vi "InspectExecuteCleanup.vi"(6 "Error":errorcluster, 7 "Actor":refnum<class "Actor.lvclass">, 9 "PreInspectExecuteError":errorcluster, 10 "Msg":T1 {"MsgAttribs"."AbsoluteTime" format="%<%x %.3X>T"}, 11 "Actor":T6) -> (2 "Msg":T1 {"MsgAttribs"."AbsoluteTime" format="%<%x %.3X>T"}, 3 "Actor":T6, 4 "Error":errorcluster, 5 "Actor":refnum<class "Actor.lvclass">)   [LabVIEW 2020, in "_Template.lvlib" / "{{Actor}}.lvlib" / "Actor.lvclass"]
uses:
  Actor.lvclass
  jettl/jettl/Metadata/Metadata.lvclass
  jettl/jettl/Msg/Msg.lvclass
  Actor.lvclass/Actor.ctl
  jettl/jettl/Actor/Actor.lvclass
  jettl/jettl/Origin.ctl
  jettl/jettl/jettl.lvlib
  jettl/jettl/Lifecycle.ctl
  jettl/jettl/MsgExecuteType.ctl
  jettl/jettl/MsgAttribs.ctl
  jettl/jettl/Msg.ctl
  jettl/jettl/PostSetup.ctl
  jettl/jettl/PreSetup.ctl
  jettl/jettl/MsgNames.ctl
  jettl/jettl/ActorAttribs.ctl
  jettl/jettl/ChildActors.ctl
  jettl/jettl/Actor.ctl
panel:
  # "This front panel should not be manipulated."
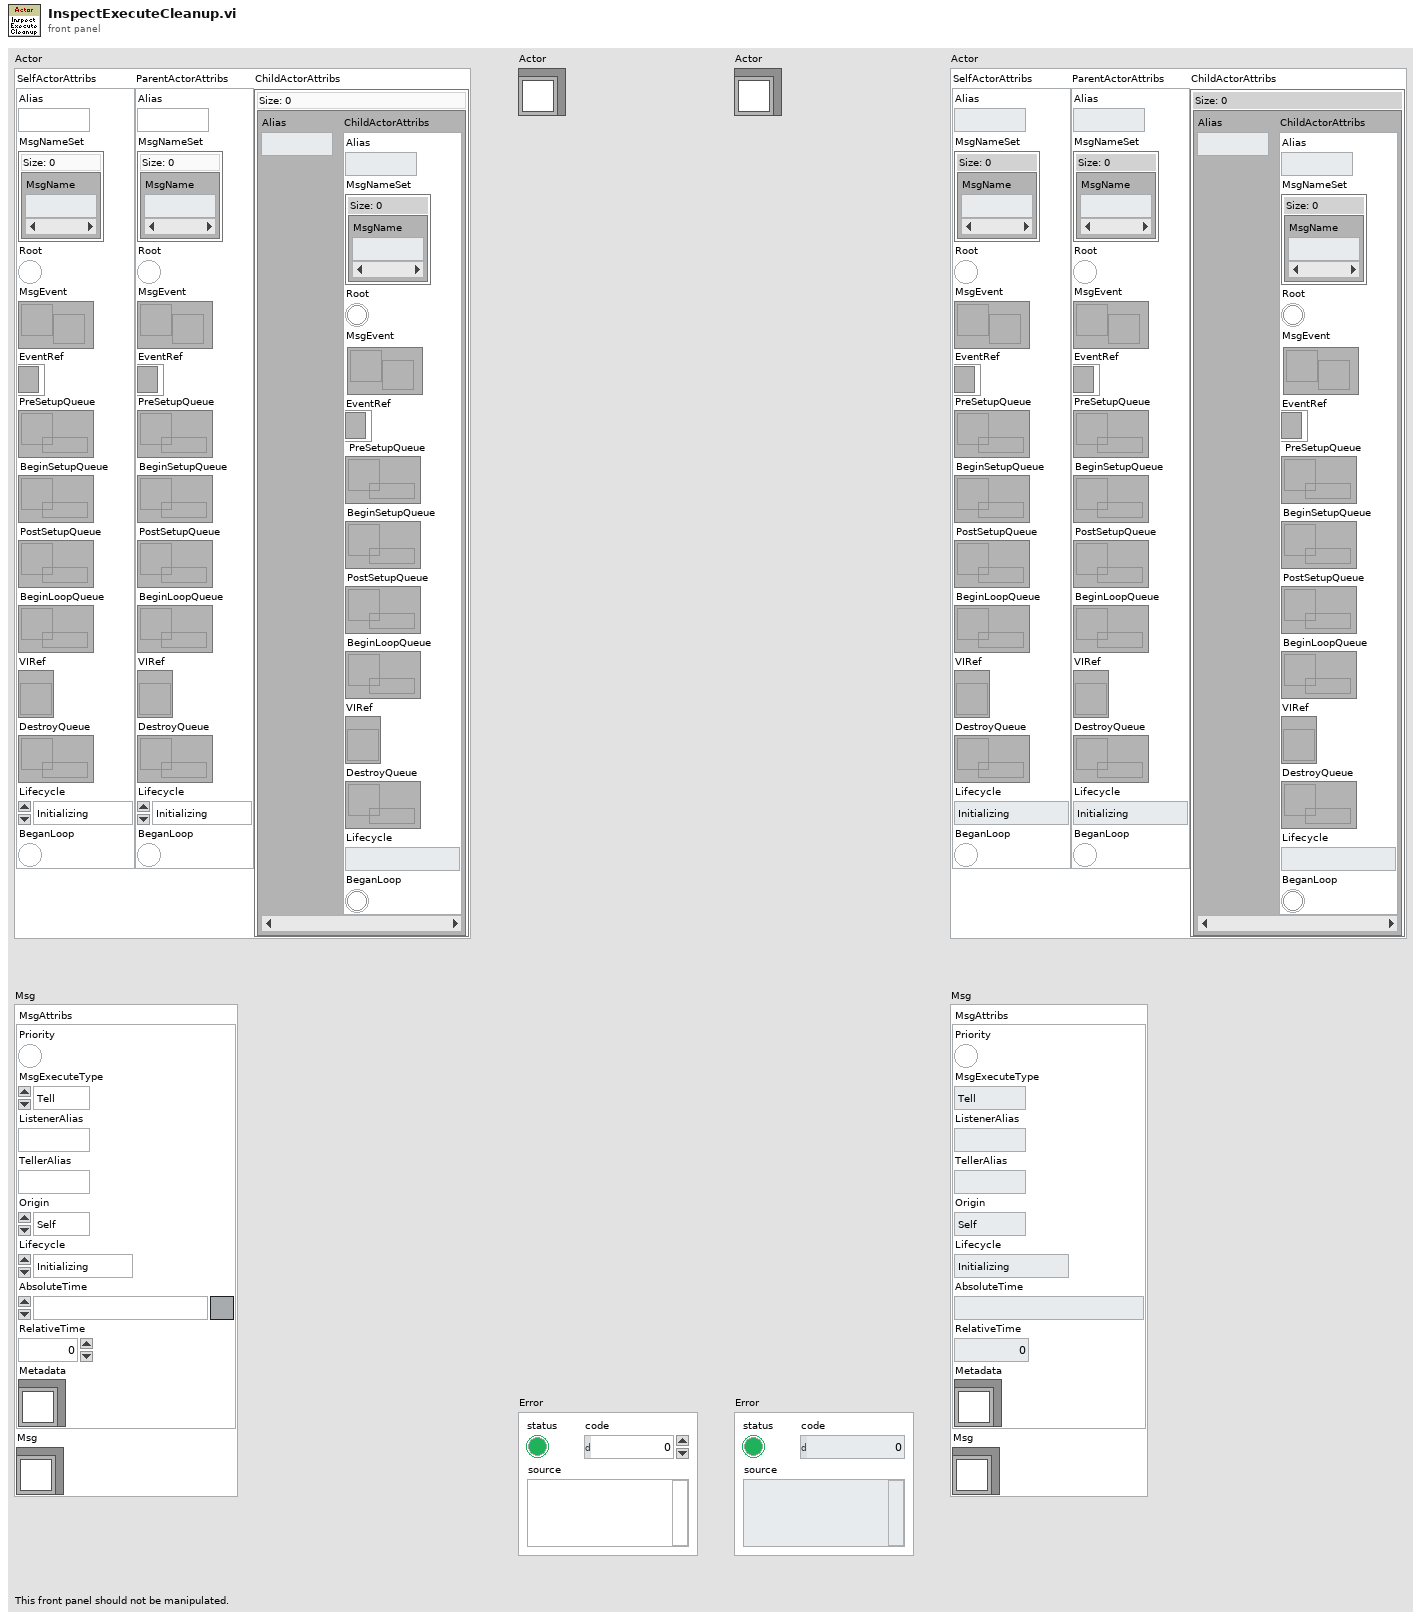
[diagram p1: front panel]
types:
  T1 = typedef "jettl.lvlib/Msg.ctl" = cluster{"MsgAttribs":T2, "Msg":refnum<class "Msg.lvclass">}
  T2 = typedef "jettl.lvlib/MsgAttribs.ctl" = cluster{"Priority":bool, "MsgExecuteType":T3, "ListenerAlias":string, "TellerAlias":string, "Origin":T4, "Lifecycle":T5, "AbsoluteTime":timestamp, "RelativeTime":dbl, "Metadata":refnum<class "Metadata.lvclass">}
  T3 = typedef "jettl.lvlib/MsgExecuteType.ctl" = enum16{"Tell", "Call"}
  T4 = typedef "jettl.lvlib/Origin.ctl" = enum16{"Self", "Parent", "Child"}
  T5 = typedef "jettl.lvlib/Lifecycle.ctl" = enum16{"Initializing", "SettingUp", "Starting", "Running", "Stopping", "TearingDown", "Terminated"}
  T6 = typedef "jettl.lvlib/Actor.ctl" = cluster{"SelfActorAttribs":T7, "ParentActorAttribs":T7, "ChildActorAttribs":T9}
  T7 = typedef "jettl.lvlib/ActorAttribs.ctl" = cluster{"Alias":string, "MsgNameSet":T8, "Root":bool, "MsgEvent":refnum<user-event>, "EventRef":refnum<event-registration>, "PreSetupQueue":refnum<queue>, "BeginSetupQueue":refnum<queue>, "PostSetupQueue":refnum<queue>, "BeginLoopQueue":refnum<queue>, "VIRef":refnum<vi>, "DestroyQueue":refnum<queue>, "Lifecycle":T5, "BeganLoop":bool}
  T8 = typedef "jettl.lvlib/MsgNames.ctl" = set{string}
  T9 = typedef "jettl.lvlib/ChildActors.ctl" = map{string, T7}
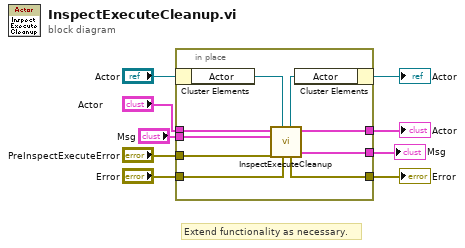
[diagram p0: block diagram]
diagram:
  # "Extend functionality as necessary."
  n1 = in-place {
    in-place-border: "Actor" -> [w16]
    in-place-border: [w15] -> w6
    in-place-border: "Error" -> [w14]
    in-place-border: "PreInspectExecuteError" -> [w10]
    in-place-border: [w13] -> w3
    in-place-border: "Msg" -> [w12]
    in-place-border: [w11] -> w1
    n2 = in-place-cluster #1("Actor") -> ("Actor"=w18:refnum<class "Actor.lvclass">)
    n3 = call-dynamic "InspectExecuteCleanup.vi"("Error"=w14, 7:"Actor"=w18, "PreInspectExecuteError"=w10, "Msg"=w12, 11:"Actor"=w16) -> ("Msg"=w11:T1, 3:"Actor"=w13:T6, "Error"=w15:errorcluster, 5:"Actor"=w17:refnum<class "Actor.lvclass">)  [unwired: 3 in]
    n4 = in-place-cluster #1("Actor"=w17) -> (→"Actor":refnum<class "Actor.lvclass">)
  }
  "Error" <- w6
  "Actor" <- w3
  "Msg" <- w1
